vi "Station_ID_Dbase.vi"() -> ()   [LabVIEW 2013]
panel:
  in  "Station ID":i32
  in  "Database name":string
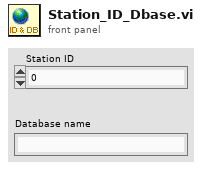
[diagram p1: front panel]
diagram:
